vi "Scores.vi"(7 "G":i32[][](array[numeric]), 9 "From":T1, 10 "Position":T2, 11 "Puzzle 15-1":T3) -> (0 "In Bounds":bool, 1 "F(n)":i32, 2 "G(n)":i32, 3 "H(n)":i32)   [LabVIEW 2020]
uses:
  Puzzle 15-1.ctl
  Position.ctl
  Dir.ctl
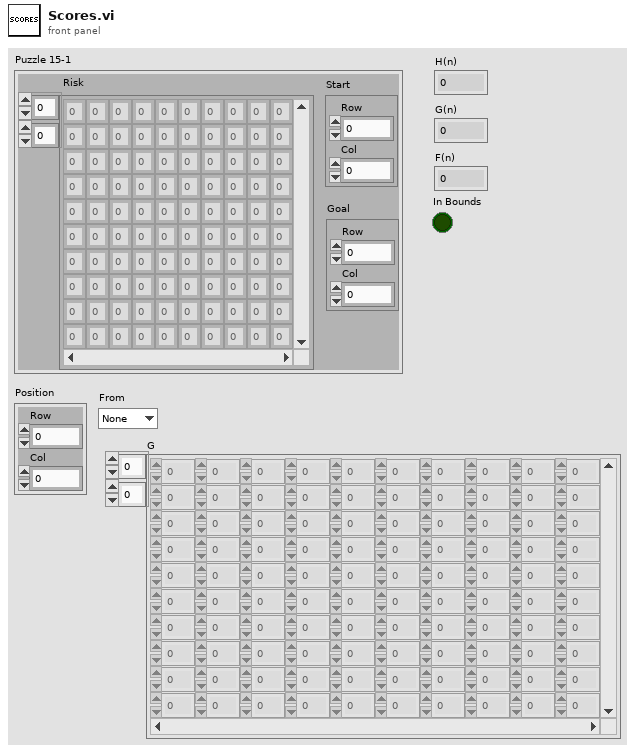
[diagram p1: front panel]
types:
  T1 = typedef "Dir.ctl" = enum16{"None", "Up", "Left", "Down", "Right"}
  T2 = typedef "Position.ctl" = cluster{"Row":i32, "Col":i32}
  T3 = typedef "Puzzle 15-1.ctl" = cluster{"Risk":i32[][], "Start":T2, "Goal":T2}
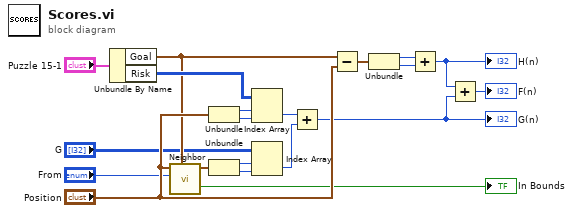
[diagram p0: block diagram]
diagram:
  n1 = Unbundle By Name("Puzzle 15-1") -> ("Goal"=w6:T2, "Risk"=w19:i32[][])
  n2 = call "Neighbor.vi"("Goal"=w6, "Dir"="From", "Position"="Position") -> ("Neighbor"=w18:T2, "In Bounds"=→"In Bounds":bool)  [unwired: 7 in]
  n3 = Unbundle("Position") -> ("Row"=w17:i32, "Col"=w16:i32)
  n4 = Unbundle(w18) -> ("Row"=w4:i32, "Col"=w3:i32)
  n5 = Index Array(array=w19, index (row)=w17, index (col)=w16) -> (element=w15:i32)
  n6 = Index Array(array="G", index (row)=w4, index (col)=w3) -> (element=w1:i32)
  n7 = Add(x=w15, y=w1) -> (x+y=w9:i32)
  "G(n)" <- w9
  n8 = Subtract(x=w6, y="Position") -> (x-y=w13:T2)
  n9 = Unbundle(w13) -> ("Row"=w12:i32, "Col"=w11:i32)
  n10 = Add(x=w12, y=w11) -> (x+y=w10:i32)
  "H(n)" <- w10
  n11 = Add(x=w10, y=w9) -> (x+y=→"F(n)":i32)
